vi "TcpClient.vi"(4 "WriteTimeout [ms] (5000)":i32=5000, 6 "ReadTimeout [ms] (5000)":i32=5000, 7 "ReadMode (Standard)":T1(ring), 8 "error in (no error)":errorcluster, 9 "OpenTimeout [ms] (5000)":i32=5000, 10 "Port":u16, 11 "Address (127.0.0.1)":string="127.0.0.1") -> (0 "error out":errorcluster, 3 "TcpClient":refnum<class "TcpClient.lvclass">)   [LabVIEW 2021, in "TcpClient.lvlib" / "TcpClient.lvclass"]
uses:
  TcpClient.lvclass
  TcpClient.lvclass/TcpClient.ctl
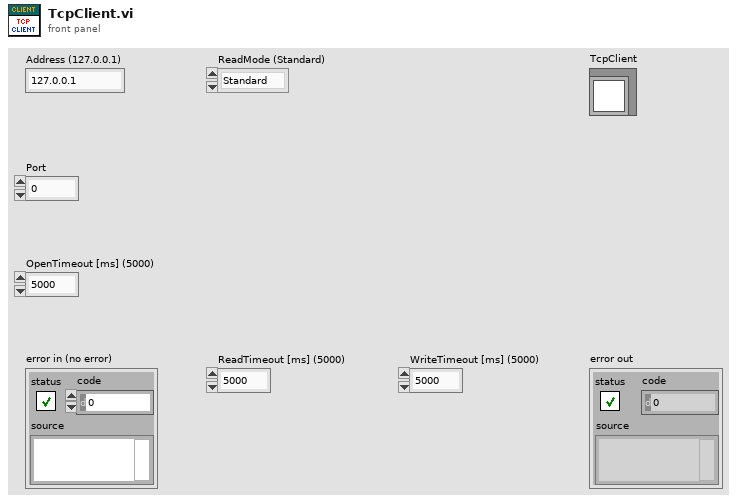
[diagram p1: front panel]
types:
  T1 = enum16{"Standard", "Buffered", "CRLF", "Immediate"}
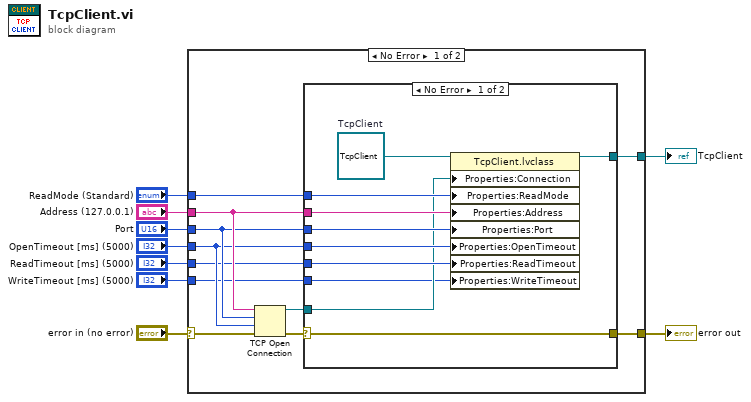
[diagram p0: block diagram]
diagram:
  n1 = case shown="No Error" "error in (no error)" {
    selector: "error in (no error)" -> [w20 w32]
    tunnel: [w14 w32] -> w8
    tunnel: "Address (127.0.0.1)" -> [w18 _]
    tunnel: "Port" -> [w17 _]
    tunnel: [w16 _] -> w5
    tunnel: "OpenTimeout [ms] (5000)" -> [w13 _]
    tunnel: "ReadMode (Standard)" -> [w12 _]
    tunnel: "WriteTimeout [ms] (5000)" -> [w11 _]
    tunnel: "ReadTimeout [ms] (5000)" -> [w10 _]
    frame No Error {
      n2 = TCP Open Connection(address=w18, remote port or service name=w17, timeout ms (60000)=w13, error in (no error)=w20) -> (connection ID=w19:refnum<k5>, error out=w15:errorcluster)  [unwired: 1 in]
      n3 = case shown="No Error" w15 {
        selector: w15 -> [w29 w31]
        tunnel: w19 -> [w23 _]
        tunnel: w18 -> [w27 _]
        tunnel: w17 -> [w26 _]
        tunnel: [w21 _] -> w16
        tunnel: [w29 w31] -> w14
        tunnel: w13 -> [w25 _]
        tunnel: w12 -> [w28 _]
        tunnel: w11 -> [w22 _]
        tunnel: w10 -> [w24 _]
        frame No Error {
          w30 = refnum<class "TcpClient.lvclass"> refnum  # TcpClient
          n4 = property class="TcpClient.lvclass"(reference=w30, "Properties:Connection"=w23, "Properties:ReadMode"=w28, "Properties:Address"=w27, "Properties:Port"=w26, "Properties:OpenTimeout"=w25, "Properties:ReadTimeout"=w24, "Properties:WriteTimeout"=w22) -> (reference out=w21:refnum<class "TcpClient.lvclass">)  [unwired: 1 in, 1 out]
        }
        frame Error {
        }
      }
    }
    frame Error {
    }
  }
  "error out" <- w8
  "TcpClient" <- w5
